vi "{{Message}}.vi"(6 "Error":errorcluster, 7 "ActorMessage":refnum<class "ActorMessage.lvclass">, 11 "Message":refnum<class "Message.lvclass">) -> (3 "Message":refnum<class "Message.lvclass">, 4 "Error":errorcluster, 5 "ActorMessage":refnum<class "ActorMessage.lvclass">)   [LabVIEW 2020, in "_Template.lvlib" / "{{Message}}.lvlib" / "ActorMessage.lvclass"]
uses:
  ActorMessage.lvclass
  Message/Message.lvclass
panel:
  # "This front panel should not be manipulated."
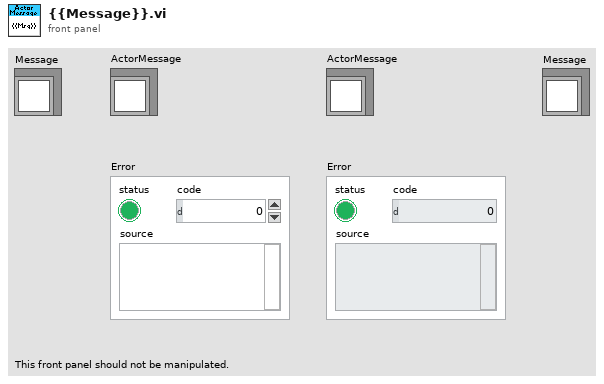
[diagram p1: front panel]
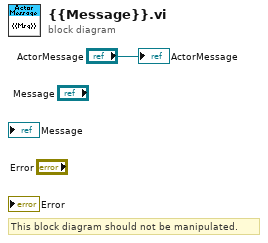
[diagram p0: block diagram]
diagram:
  # "This block diagram should not be manipulated."
  "ActorMessage" <- "ActorMessage"
